vi "GetDigitalInputProperties.vi"(11 "channel properties":T2[](array[typedef])) -> (3 "tdms properties":T1[](array[typedef]))   [LabVIEW 2017, in "Tdms.lvlib"]
uses:
  <vilib>/addons/InsightCM/Utilities/Tdms/Tdms.lvlib
  <vilib>/addons/InsightCM/MessageBus/Base/controls/KeyValuePair.ctl
  <vilib>/addons/InsightCM/Utilities/Tdms/controls/Property.ctl
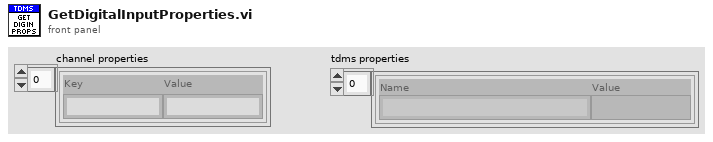
[diagram p1: front panel]
types:
  T1 = typedef "Tdms.lvlib/Property.ctl" = cluster{"Name":string, "Value":variant}
  T2 = typedef "KeyValuePair.ctl" = cluster{"Key":string, "Value":string}
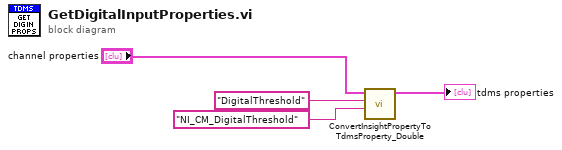
[diagram p0: block diagram]
diagram:
  n1 = call <vilib>:"ConvertInsightPropertyToTdmsProperty_Double.vi"("Tdms Property Name"="NI_CM_DigitalThreshold" ("Name"), "Insight Property Name"="DigitalThreshold" ("Name"), "Insight Properties"="channel properties") -> ("Tdms Properties"=→"tdms properties":T1[])  [unwired: 8 in]
